vi "prc_SetPackaged.vi"(8 "error in":errorcluster, 10 "string":string, 11 "SQL query":string="prc_SetPackaged") -> (0 "error out":errorcluster, 2 "Array":string[][](array[string]))   [LabVIEW 2013]
uses:
  <vilib>/addons/database/Connection.llb/DB Tools Open Connec (String).vi
  <vilib>/addons/database/Connection.llb/Conn Execute.vi
  <vilib>/addons/database/Recordset.llb/Rec Fetch Recordset Data (R).vi
  <vilib>/addons/database/Recordset.llb/Rec Destroy - Connection.vi
  <vilib>/addons/database/NI_Database_API.lvlib
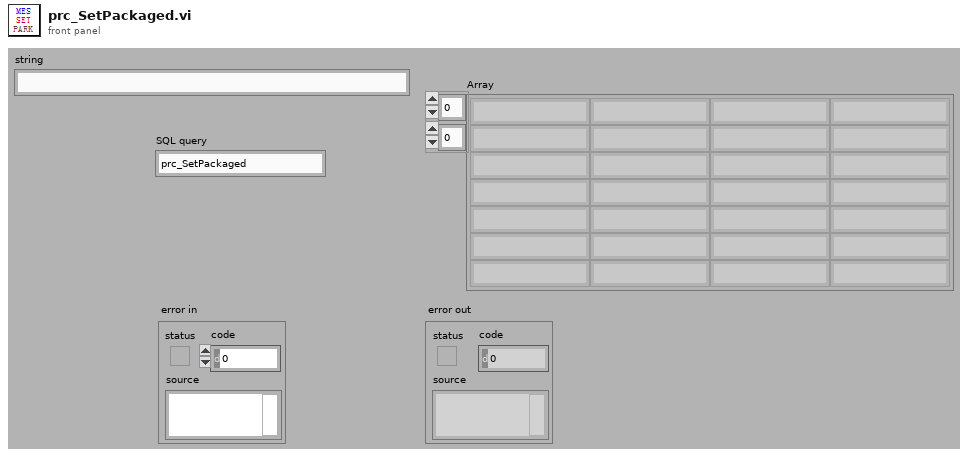
[diagram p1: front panel]
types:
  T1 = typedef "NI_Database_API.lvlib/Conn ObjectReference.ctl" = refnum<k1>
  T2 = typedef "NI_Database_API.lvlib/Rec ObjectReference.ctl" = refnum<k1>
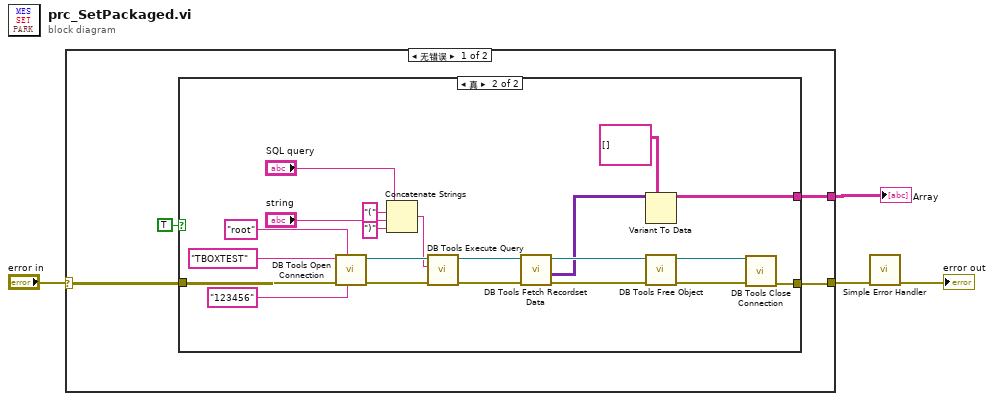
[diagram p0: block diagram]
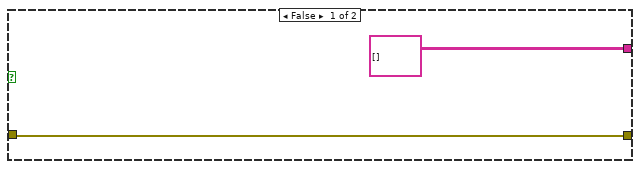
[diagram p2: hidden frame]
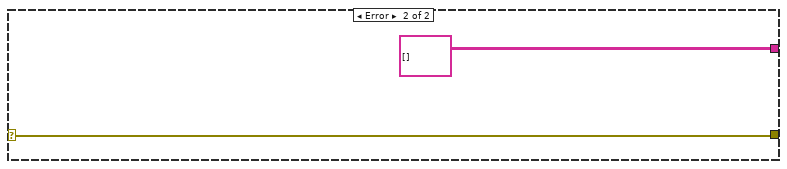
[diagram p3: hidden frame]
diagram:
  n1 = case shown="无错误" "error in" {
    selector: "error in" -> [w6 w33]
    tunnel: [w8 w33] -> w4
    tunnel: [w7 string[][] []] -> w1
    frame No Error {
      n2 = case shown="真" TRUE {
        tunnel: [w10 w25] -> w8
        tunnel: [string[][] [] w18] -> w7
        tunnel: w6 -> [w10 w17]
        frame False {
        }
        frame True {
          n3 = call-poly <vilib>:"DB Tools Open Connection.vi"("password"="123456", "userID"="root", "error in (no error)"=w17, "connection information"="TBOXTEST") -> ("error out"=w29:errorcluster, "connection reference"=w28:T1)  [unwired: 4 in]
          n4 = Concatenate Strings("SQL query", "(" ("字符串"), "string", ")" ("字符串")) -> (w11:string)
          n5 = call-poly <vilib>:"DB Tools Execute Query.vi"("error in (no error)"=w29, "SQL query"=w11, "connection reference"=w28) -> ("error out"=w26:errorcluster, "recordset reference"=w27:T2)  [unwired: 5 in]
          n6 = call-poly <vilib>:"DB Tools Fetch Recordset Data.vi"("error in (no error)"=w26, "recordset reference"=w27) -> ("error out"=w24:errorcluster, "recordset data"=w20:variant[][], "recordset reference out"=w23:T2)  [unwired: 3 in]
          n7 = Variant To Data(type=string[][] [], Variant=w20) -> (data=w18:string[][])  [unwired: 1 in, 1 out]
          n8 = call-poly <vilib>:"DB Tools Free Object.vi"("error in (no error)"=w24, "recordset reference"=w23) -> ("error out"=w22:errorcluster, "connection reference"=w21:T1)  [unwired: 8 in]
          n9 = call <vilib>:"DB Tools Close Connection.vi"("error in (no error)"=w22, "connection reference"=w21) -> ("error out"=w25:errorcluster)  [unwired: 5 in]
        }
      }
    }
    frame Error {
    }
  }
  "Array" <- w1
  n10 = call <vilib>:"Simple Error Handler.vi"("error in (no error)"=w4) -> ("error out"=→"error out":errorcluster)  [unwired: 4 in, 4 out]
